vi "InitDH.vi"(8 "error in (no error)":errorcluster, 11 "DataHandler in":refnum<class "DataHandler.lvclass">) -> (0 "error out":errorcluster, 3 "DataHandler out":refnum<class "DataHandler.lvclass">)   [LabVIEW 2017, in "DataHandler.lvclass"]
uses:
  DataHandler.lvclass
  DataHandler.lvclass/DataHandler.ctl
  <vilib>/drjdpowell/SQLite Library/SQL Connection/Execute SQL (Single Integer).vi
  <vilib>/drjdpowell/SQLite Library/SQLite.lvlib
  <vilib>/drjdpowell/SQLite Library/SQL Connection/Connection.lvclass
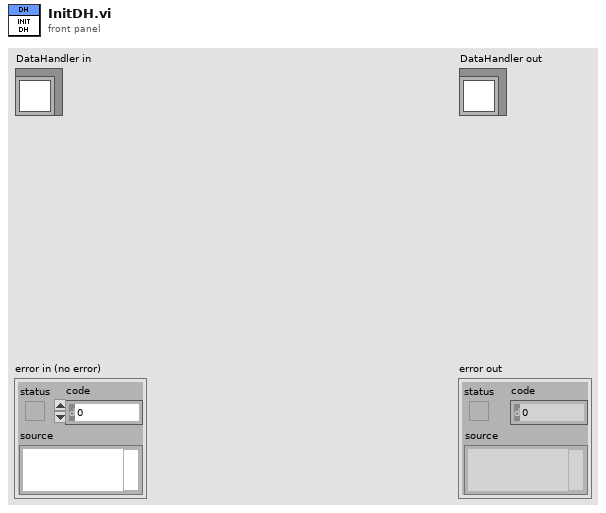
[diagram p1: front panel]
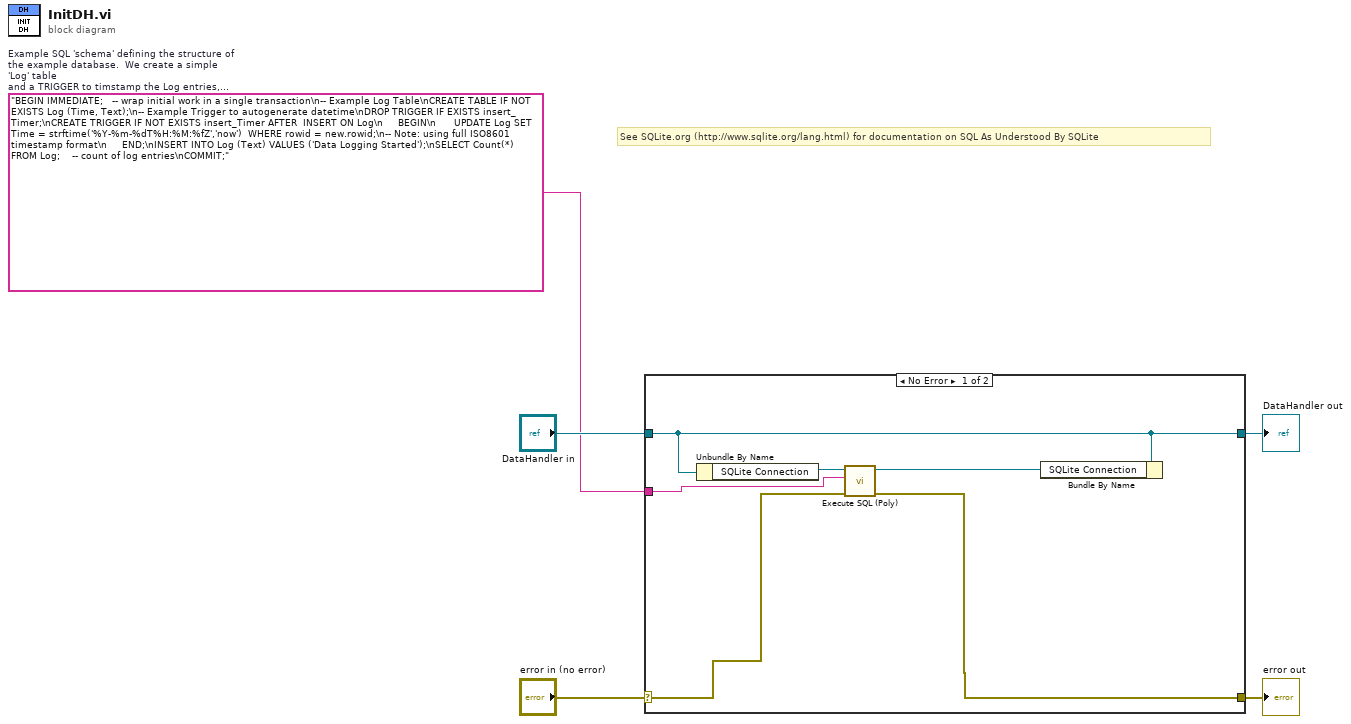
[diagram p0: block diagram]
diagram:
  w1 = "BEGIN IMMEDIATE;   -- wrap initial work in a single transaction\n-- Example Log Table\nCREATE TABLE IF NOT EXISTS Log (Time, Text);\n-- Example Trigger to autogenerate datetime\nDROP TRIGGER IF EXISTS insert_Timer;\nCREATE TRIGGER IF NOT EXISTS insert_Timer AFTER  INSERT ON Log\n     BEGIN\n      UPDATE Log SET Time = strftime('%Y-%m-%dT%H:%M:%fZ','now')  WHERE rowid = new.rowid;\n-- Note: using full ISO8601 timestamp format\n     END;\nINSERT INTO Log (Text) VALUES ('Data Logging Started');\nSELECT Count(*) FROM Log;    -- count of log entries\nCOMMIT;"  # Example SQL 'schema' defining the structure of the example database.  We create a simple 'Log' table and a TRIGGER to timstamp the Log entries, then a simple 'Data' table
  # "See SQLite.org (http://www.sqlite.org/lang.html) for documentation on SQL As Understood By SQLite"
  n1 = case shown="No Error" "error in (no error)" {
    selector: "error in (no error)" -> [w9 w13]
    tunnel: [w8 w13] -> w4
    tunnel: [w7 w12] -> w2
    tunnel: "DataHandler in" -> [w7 w12]
    tunnel: w1 -> [w6 _]
    frame No Error {
      n2 = Unbundle By Name(w7) -> ("SQLite Connection"=w11:refnum<class "Connection.lvclass">)
      n3 = call-poly <vilib>:"Execute SQL (Poly).vi"("error in (no error)"=w9, "SQL"=w6, "SQLite Connection in"=w11) -> ("error out"=w8:errorcluster, "SQLite Connection out"=w10:refnum<class "Connection.lvclass">)  [unwired: 6 in, 1 out]
      n4 = Bundle By Name(cluster=w7, "SQLite Connection"=w10) -> ()  [unwired: 1 out]
    }
    frame Error {
    }
  }
  "error out" <- w4
  "DataHandler out" <- w2
